vi "test-FlyWheel-Sim-Test2.vi"() -> (3 "All Passed":bool)   [LabVIEW 2019]
uses:
  <vilib>/Rock Robotics/WPI/ThirdParty/JAS_Junk/TrajLib/DCMOTOR_TYPES_ENUM.ctl
  <vilib>/Analysis/Matrix/Datatypes/RealMatrix.ctl
  <vilib>/Rock Robotics/WPI/ThirdParty/JAS_Junk/TrajLib/DCMotor_GetCIM.vi
  <vilib>/Rock Robotics/WPI/ThirdParty/JAS_Junk/TrajLib/DCMotor_GetAndymark9015.vi
  <vilib>/Rock Robotics/WPI/ThirdParty/JAS_Junk/TrajLib/DCMotor_GetAndymarkRs775_125.vi
  <vilib>/Rock Robotics/WPI/ThirdParty/JAS_Junk/TrajLib/DCMotor_GetBag.vi
  <vilib>/Rock Robotics/WPI/ThirdParty/JAS_Junk/TrajLib/DCMotor_GetBanebotsRs550.vi
  <vilib>/Rock Robotics/WPI/ThirdParty/JAS_Junk/TrajLib/DCMotor_GetBanebotsRs775.vi
  <vilib>/Rock Robotics/WPI/ThirdParty/JAS_Junk/TrajLib/DCMotor_GetFalcon500.vi
  <vilib>/Rock Robotics/WPI/ThirdParty/JAS_Junk/TrajLib/DCMotor_GetMiniCIM.vi
  <vilib>/Rock Robotics/WPI/ThirdParty/JAS_Junk/TrajLib/DCMotor_GetNEO.vi
  <vilib>/Rock Robotics/WPI/ThirdParty/JAS_Junk/TrajLib/DCMotor_GetNEO550.vi
  <vilib>/Rock Robotics/WPI/ThirdParty/JAS_Junk/TrajLib/DCMotor_GetRomiBuiltIn.vi
  <vilib>/Rock Robotics/WPI/ThirdParty/JAS_Junk/TrajLib/DCMotor_GetVex775Pro.vi
  <vilib>/Rock Robotics/WPI/ThirdParty/JAS_Junk/TrajLib/PIDController_Calculate_SP_PV.vi
  <vilib>/Rock Robotics/WPI/ThirdParty/JAS_Junk/TrajLib/PIDController_AtSetpoint.vi
  <vilib>/Rock Robotics/WPI/ThirdParty/JAS_Junk/TrajLib/PIDController_SetPID.vi
  <vilib>/Rock Robotics/WPI/ThirdParty/JAS_Junk/TrajLib/PIDController_SetIntegratorRange.vi
  <vilib>/Rock Robotics/WPI/ThirdParty/JAS_Junk/TrajLib/PIDController_SetTolerancePandV.vi
  <vilib>/Rock Robotics/WPI/ThirdParty/JAS_Junk/TrajLib/PIDController_DisableContinousInput.vi
  <vilib>/Rock Robotics/WPI/ThirdParty/JAS_Junk/TrajLib/PIDController_EnableContinousInput.vi
  <vilib>/Rock Robotics/WPI/ThirdParty/JAS_Junk/TrajLib/PIDController_Reset.vi
  <vilib>/Rock Robotics/WPI/ThirdParty/JAS_Junk/TrajLib/PIDController_NewPeriod.vi
  <vilib>/Rock Robotics/WPI/ThirdParty/JAS_Junk/TrajLib/BatterySim_CalculateLoadedBatteryVoltage.vi
  <vilib>/Rock Robotics/WPI/ThirdParty/JAS_Junk/TrajLib/DCMotor_New.vi
  <vilib>/Rock Robotics/WPI/ThirdParty/JAS_Junk/TrajLib/Units_RotationsPerMinuteToRadiansPerSecond.vi
  <vilib>/Rock Robotics/WPI/ThirdParty/JAS_Junk/TrajLib/PIDController_SetSetpoint.vi
  <vilib>/Rock Robotics/WPI/ThirdParty/JAS_Junk/TrajLib/PIDController_Calculate_PV.vi
  <vilib>/Rock Robotics/WPI/ThirdParty/JAS_Junk/TrajLib/ControllerUtil_GetModulusError.vi
  <vilib>/Rock Robotics/SystemInterfaces/NetworkCommunication/NetComm_UsageReport_report.vi
  <vilib>/Rock Robotics/WPI/ThirdParty/JAS_Junk/TrajLib/Util_LibraryGlobals.vi
  <vilib>/Rock Robotics/WPI/ThirdParty/JAS_Junk/TrajLib/Trajectory_Library.lvlib
  <vilib>/Analysis/Matrix/NI_Matrix.lvlib
panel:
  out "Speed Control Passed":bool
  out "Speed Ctrl":T1(graph)
  out "Error":bool
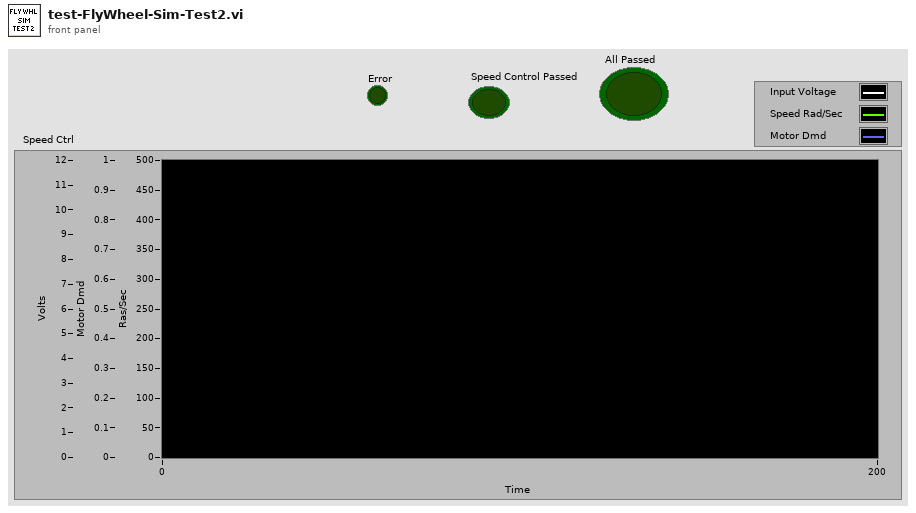
[diagram p1: front panel]
types:
  T1 = cluster{dbl, "Velocity_RadPerSec":dbl, "upper limit":dbl}
  T2 = typedef "NI_Matrix.lvlib/RealMatrix.ctl" = dbl[][]
  T3 = typedef "Trajectory_Library.lvlib/DCMOTOR_TYPES_ENUM.ctl" = enum16{"CIM", "AndyMark 9015", "Andy Mark RS 775 125", "Bag", "BaneBots RS 550", "BaneBots RS 775", "Falcon 500", "Mini CIM", "NEO", "NEO 550", "Romi BuiltIn", "Vex 775 Pro"}
  T4 = typedef "Trajectory_Library.lvlib/DCMOTOR.CTL" = cluster{"nominalVoltage_Volts":dbl, "StallTorque_NM":dbl, "StallCurrent_Amps":dbl, "FreeCurrent_Amps":dbl, "FreeSpeed_RadPerSec":dbl, "R_Ohms":dbl, "KvINV_RadPerSecPerVolt":dbl, "Kt_NMPerAmp":dbl, "L_H":dbl, "Jr_KgM2":dbl}
  T5 = typedef "Trajectory_Library.lvlib/FLYWHEEL_SIM.ctl" = cluster{"LinearSystemSim":T6, "GearBox":T4, "Gearing":dbl}
  T6 = typedef "Trajectory_Library.lvlib/LINEAR_SYSTEM_SIM.ctl" = cluster{"m_Plant":T7, "m_X":T2, "m_Y":T2, "m_U":T2, "MeasureStdDev":T2}
  T7 = typedef "Trajectory_Library.lvlib/LINEAR_SYSTEM.ctl" = cluster{"m_A":T2, "m_B":T2, "m_C":T2, "m_D":T2, "States":i32, "Inputs":i32, "Outputs":i32}
  T8 = typedef "Trajectory_Library.lvlib/PID_TUNING.ctl" = cluster{"Kp":dbl, "Ki":dbl, "Kd":dbl, "MaximumIntegral":dbl, "MinimumIntegral":dbl}
  T9 = typedef "Trajectory_Library.lvlib/PID_INPUT_LIMITS.ctl" = cluster{"MaxInput":dbl, "MinInput":dbl, "Continuous":bool}
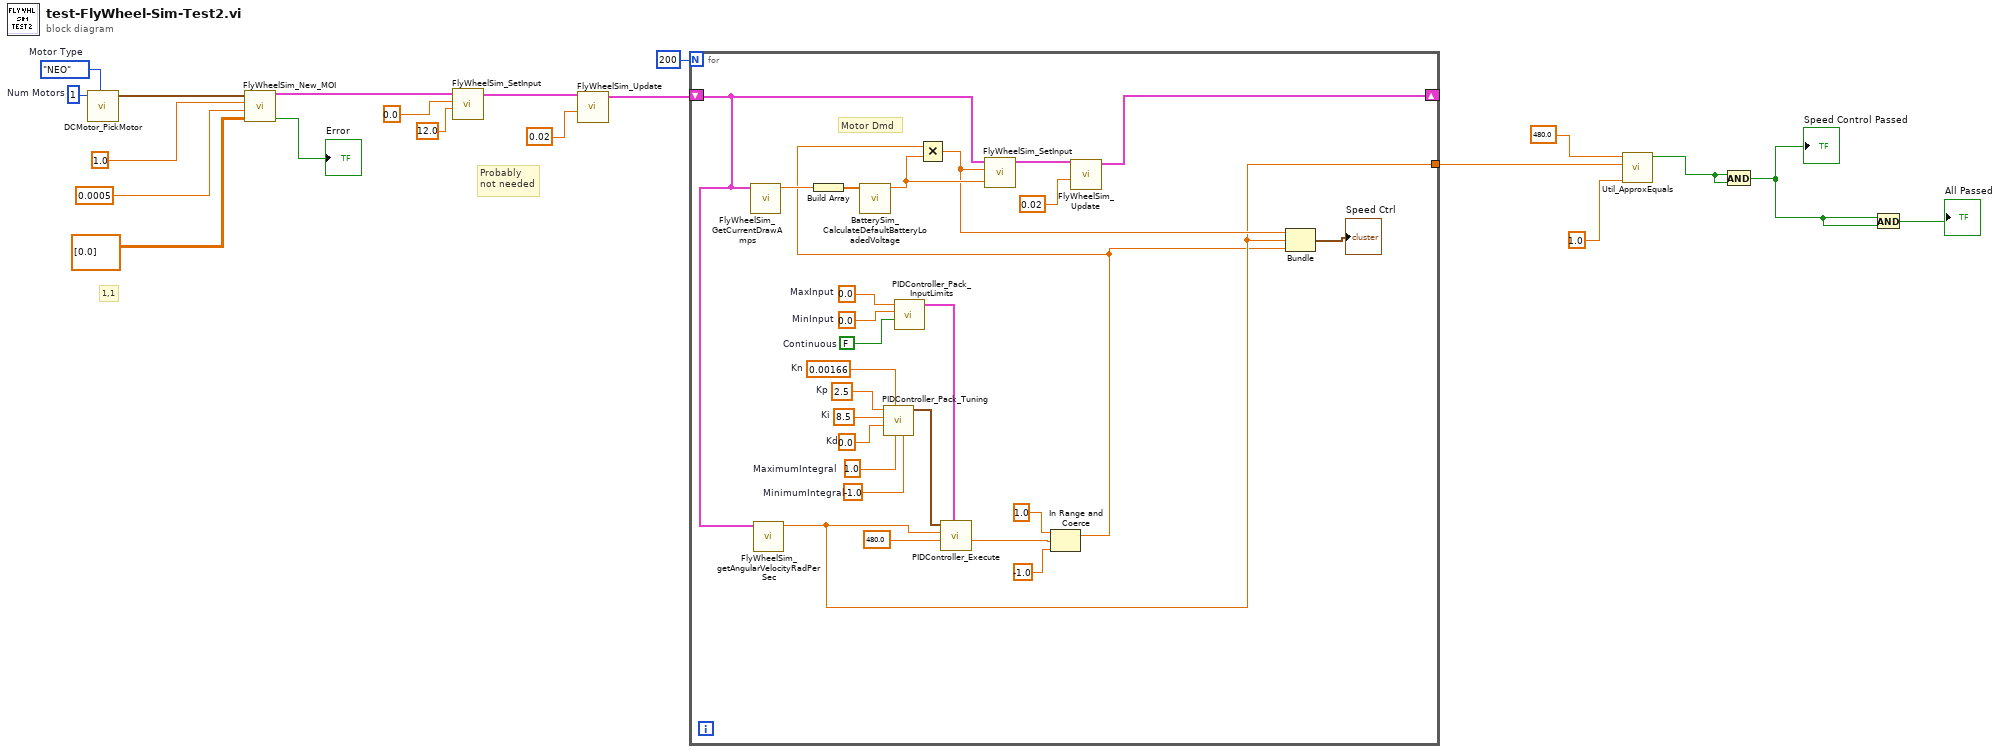
[diagram p0: block diagram]
diagram:
  w20 = 1  # Num Motors
  w19 = DCMOTOR_TYPES_ENUM."NEO"  # Motor Type
  # "Probably \nnot needed"
  # "1,1"
  n1 = call <vilib>:"DCMotor_PickMotor.vi"("DCMOTOR_TYPES"=w19, "Num Motors"=w20) -> ("DCMOTOR"=w7:T4)  [unwired: 9 in]
  n2 = call <vilib>:"FlyWheelSim_New_MOI.vi"("MeasurementStdDev"=T2 [[0.0]], "jKgMetersSquared"=0.0005, "Gearing"=1.0, "GearBox"=w7) -> ("Error"=→"Error":bool, "FlyWheelSim"=w13:T5)  [unwired: 6 in]
  n3 = call <vilib>:"FlyWheelSim_SetInput.vi"("Battery_Volts"=12.0, "Volts"=0.0, "FlyWheelSim"=w13) -> ("out FlyWheelSim"=w9:T5)  [unwired: 8 in]
  n4 = call <vilib>:"FlyWheelSim_Update.vi"("dT_Seconds"=0.02, "FlyWheelSim"=w9) -> ("out FlyWheelSim"=w8:T5)  [unwired: 8 in, 1 out]
  n5 = for {
    N: 200 -> [_]
    shift-right: [w39] -> _
    shift-left: w8 -> [w26]
    tunnel: [w22] -> w2
    w38 = 0.00166  # Kn
    w37 = 0.0  # MaxInput
    w36 = 0.0  # MinInput
    w35 = FALSE  # Continuous
    w34 = 2.5  # Kp
    w33 = 8.5  # Ki
    w32 = 0.0  # Kd
    w31 = 1.0  # MaximumIntegral
    w30 = -1.0  # MinimumIntegral
    # "Motor Dmd"
    n6 = call <vilib>:"FlyWheelSim_GetCurrentDrawAmps.vi"("FlyWheelSim"=w26) -> ("Current_Amps"=w45:dbl)  [unwired: 10 in]
    n7 = call <vilib>:"FlyWheelSim_getAngularVelocityRadPerSec.vi"("FlyWheelSim"=w26) -> ("Velocity_RadPerSec"=w22:dbl)  [unwired: 10 in]
    n8 = Build Array(w45) -> (w46:dbl[])
    n9 = call <vilib>:"BatterySim_CalculateDefaultBatteryLoadedVoltage.vi"("Currents"=w46) -> ("Voltage"=w44:dbl)  [unwired: 10 in]
    n10 = call <vilib>:"PIDController_Pack_Tuning.vi"("MinimumIntegral"=w30, "MaximumIntegral"=w31, "Kn"=w38, "Kd"=w32, "Ki"=w33, "Kp"=w34) -> ("PID Tuning"=w29:T8)  [unwired: 5 in]
    n11 = call <vilib>:"PIDController_Pack_InputLimits.vi"("Continuous"=w35, "MinInput"=w36, "MaxInput"=w37) -> ("PID Input Limits"=w28:T9)  [unwired: 8 in]
    n12 = call <vilib>:"PIDController_Execute.vi"("PID Input Limits"=w28, "SP-SetPoint"=480.0, "PV-Measurement"=w22, "PID Tuning"=w29) -> ("CO-ControlOutput"=w23:dbl)  [unwired: 5 in, 2 out]
    n13 = In Range and Coerce(upper limit=1.0, x=w23, lower limit=-1.0) -> (coerced(x)=w21:dbl)  [unwired: 1 out]
    n14 = Multiply(x=w21, y=w44) -> (x*y=w40:dbl)
    n15 = call <vilib>:"FlyWheelSim_SetInput.vi"("Battery_Volts"=w44, "Volts"=w40, "FlyWheelSim"=w26) -> ("out FlyWheelSim"=w43:T5)  [unwired: 8 in]
    n16 = call <vilib>:"FlyWheelSim_Update.vi"("dT_Seconds"=0.02, "FlyWheelSim"=w43) -> ("out FlyWheelSim"=w39:T5)  [unwired: 8 in, 1 out]
    n17 = Bundle(w40, "Velocity_RadPerSec"=w22, "upper limit"=w21) -> (→"Speed Ctrl":T1)  [unwired: 1 in]
  }
  n18 = call <vilib>:"Util_ApproxEquals.vi"("Tolerance"=1.0, "Value 2"=w2, "Value 1"=480.0 ("y")) -> ("ApproxEquals"=w1:bool)  [unwired: 8 in]
  n19 = And(x=w1, y=w1) -> (x .and. y?=w3:bool)
  "Speed Control Passed" <- w3
  n20 = And(x=w3, y=w3) -> (x .and. y?=→"All Passed":bool)
